vi "Base Error Code.vi"() -> (3 "base error code":i32)   [LabVIEW 2017, in "DSF Core.lvlib"]
uses:
  DSF Core.lvlib
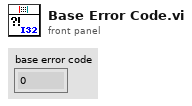
[diagram p1: front panel]
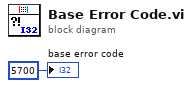
[diagram p0: block diagram]
diagram:
  "base error code" <- 5700 ("base error code")
